vi "Initialize.vi"(8 "error in (no error)":errorcluster, 9 "ID Query (T: Query)":bool=TRUE, 10 "Reset Device (T: Reset)":bool=TRUE, 11 "VISA resource name":refnum<visa-resource-name>) -> (0 "error out":errorcluster, 3 "VISA resource name out":refnum<visa-resource-name>)   [LabVIEW 2020, in "Agilent E364X Series.lvlib"]
doc: "Passes the addressing information in the instrument resource name to the VISA Open VI and returns the instrument ID.\n\nNote: \nThis instrument driver supports serial communication. If problems are encountered when using serial communication, recommend using baud rates less than 19,200 and hardware handshaking. National Instruments does not provide technical support for the oscilloscope’s physical serial interface. National Instruments will support driver related issues. If you need technical support related to the physical serial interface on either the Agilent E364xA series please contact Agilent.\n\nSettings for Serial Use, please make sure these values are set in Measurement & Automation Explorer and on the instrument. Also be sure they match exactly with each other.\n\n-Baud Rate: 300, 600, 1200, 2400, 4800, or 9600 (factory setting) \n-Parity and Data Bit : None / 8 data bits (factory setting), Even / 7 data bit , or Odd / 7 data bit \n-Number of Start Bit : 1 bit (fixed on instrument) \n-Number of Stop Bit : 2 bits (fixed on instrument) \n-Handshaking: DTR / DSR (fixed on instrument)"
uses:
  Agilent E364X Series.lvlib
panel:
  # "© 2005, National Instruments, Corporation.  All Rights Reserved."
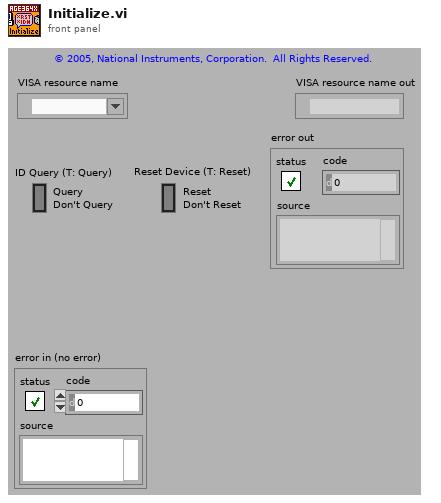
[diagram p1: front panel]
types:
  T1 = cluster{"Status":bool, "Code":i32, "Source (VI Name)":string}
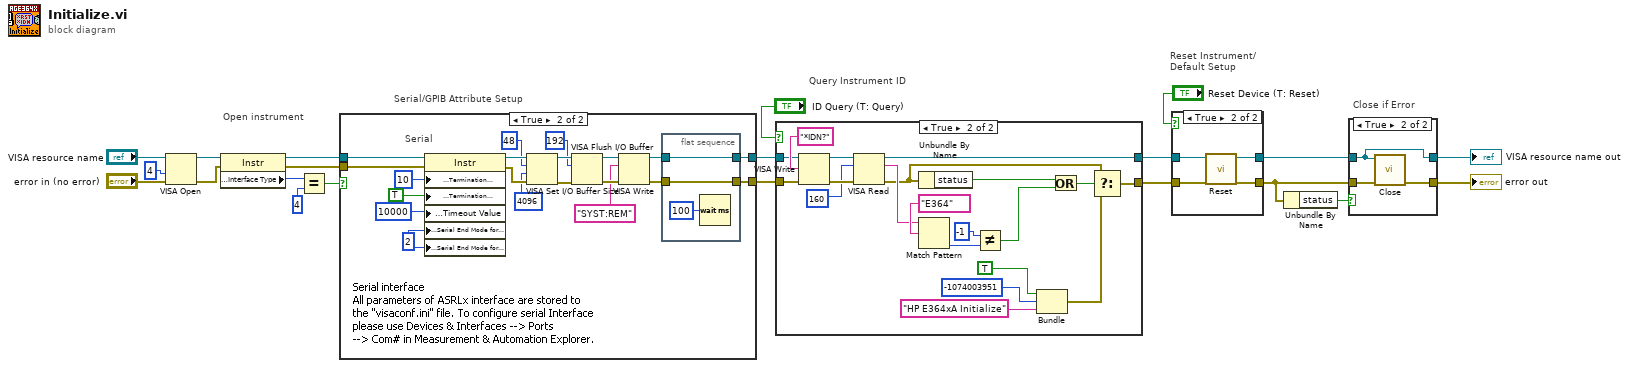
[diagram p0: block diagram]
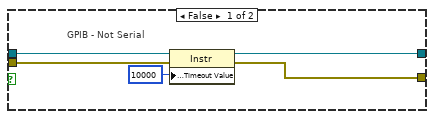
[diagram p3: hidden frame]
diagram:
  # "Serial/GPIB Attribute Setup"
  # "Close if Error"
  # "Reset Instrument/\nDefault Setup"
  # "Open instrument"
  # "Query Instrument ID"
  n1 = VISA Open(access mode=u32 4, error in (no error)="error in (no error)", VISA resource name="VISA resource name") -> (VISA resource name=w16:refnum<visa-resource-name>, error out=w17:errorcluster)  [unwired: 2 in]
  n2 = property class="Instr"(reference=w16, error in=w17) -> (reference out=w13:refnum<visa-resource-name>, error out=w14:errorcluster, "Interface Information:Interface Type"=w15:u16)
  n3 = Equal?(x=w15, y=u16 4 ("Serial")) -> (x = y?=w18:bool)
  n4 = case shown="True" w18 {
    tunnel: w13 -> [w26 w46]
    tunnel: w14 -> [w25 w45]
    tunnel: [w24 w27] -> w5
    tunnel: [w23 w29] -> w4
    frame False {
      # "GPIB - Not Serial"
      n5 = property class="Instr"(reference=w26, error in=w25, "General Settings:Timeout Value"=u32 10000) -> (reference out=w24:refnum<visa-resource-name>, error out=w23:errorcluster)
    }
    frame True {
      w34 = 2
      # "Serial"
      n6 = property class="Instr"(reference=w46, error in=w45, "Message Based Settings:Termination Character"=u8 10, "Message Based Settings:Termination Character Enable"=TRUE, "General Settings:Timeout Value"=u32 10000, "Serial Settings:Serial End Mode for Writes"=w34, "Serial Settings:Serial End Mode for Reads"=w34) -> (reference out=w44:refnum<visa-resource-name>, error out=w43:errorcluster)
      n7 = VISA Set I/O Buffer Size(VISA resource name=w44, mask (16)=u16 48, size (4096)=u32 4096 ("size (0)"), error in (no error)=w43) -> (VISA resource name out=w42:refnum<visa-resource-name>, error out=w41:errorcluster)
      n8 = VISA Flush I/O Buffer(VISA resource name=w42, mask (16)=u16 192, error in (no error)=w41) -> (VISA resource name out=w40:refnum<visa-resource-name>, error out=w39:errorcluster)
      n9 = VISA Write(VISA resource name=w40, write buffer="SYST:REM", error in (no error)=w39) -> (VISA resource name out=w28:refnum<visa-resource-name>, error out=w30:errorcluster)  [unwired: 1 out]
      n10 = flat-sequence {
        tunnel: w30 -> [w48]
        tunnel: [w48] -> w29
        tunnel: w28 -> [w47]
        tunnel: [w47] -> w27
        frame #0 {
          n11 = Wait (ms)(milliseconds to wait=u32 100) -> ()  [unwired: 1 out]
        }
      }
    }
  }
  n12 = case shown="True" "ID Query (T: Query)" {
    tunnel: [w50 w59] -> w9
    tunnel: w4 -> [w50 w63]
    tunnel: [w51 w66] -> w10
    tunnel: w5 -> [w51 w69]
    frame False {
    }
    frame True {
      n13 = VISA Write(VISA resource name=w69, write buffer="*IDN?", error in (no error)=w63) -> (VISA resource name out=w64:refnum<visa-resource-name>, error out=w68:errorcluster)  [unwired: 1 out]
      n14 = VISA Read(VISA resource name=w64, byte count=u32 160, error in (no error)=w68) -> (VISA resource name out=w66:refnum<visa-resource-name>, read buffer=w67:string, error out=w61:errorcluster)  [unwired: 1 out]
      n15 = Unbundle By Name(w61) -> ("status"=w60:bool)
      n16 = Match Pattern(string=w67, regular expression="E364") -> (offset past match=w57:i32)  [unwired: 1 in, 3 out]
      n17 = Not Equal?(x=-1, y=w57) -> (x != y?=w52:bool)
      n18 = Bundle("Status"=TRUE, "Code"=-1074003951, "Source (VI Name)"="HP E364xA Initialize") -> (w53:T1)  [unwired: 1 in]
      n19 = Or(x=w60, y=w52) -> (x .or. y?=w62:bool)
      n20 = Select(t=w61, s=w62, f=w53) -> (s? t:f=w59:T1)
    }
  }
  n21 = case shown="True" "Reset Device (T: Reset)" {
    tunnel: w9 -> [w72 w76]
    tunnel: [w72 w74] -> w11
    tunnel: w10 -> [w73 w77]
    tunnel: [w73 w75] -> w12
    frame False {
    }
    frame True {
      n22 = call "Reset.vi"("error in (no error)"=w76, "VISA resource name"=w77) -> ("error out"=w74:errorcluster, "VISA resource name out"=w75:refnum<visa-resource-name>)  [unwired: 8 in]
    }
  }
  n23 = Unbundle By Name(w11) -> ("status"=w7:bool)
  n24 = case shown="True" w7 {
    tunnel: w12 -> [w79 w80]
    tunnel: w11 -> [w78 w82]
    tunnel: [w79 w80] -> w3
    tunnel: [w78 w81] -> w2
    frame False {
    }
    frame True {
      n25 = call "Close.vi"("error in (no error)"=w82, "VISA resource name"=w80) -> ("error out"=w81:errorcluster)  [unwired: 9 in]
    }
  }
  "error out" <- w2
  "VISA resource name out" <- w3
